vi "RangeCases.vi"() -> ()   [LabVIEW 2019]
panel:
  in  "Numeric 2":u8
  in  "Numeric":u8
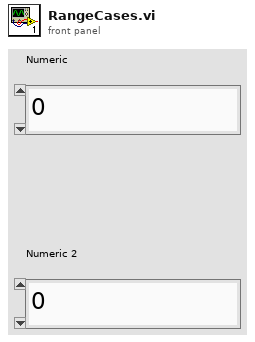
[diagram p1: front panel]
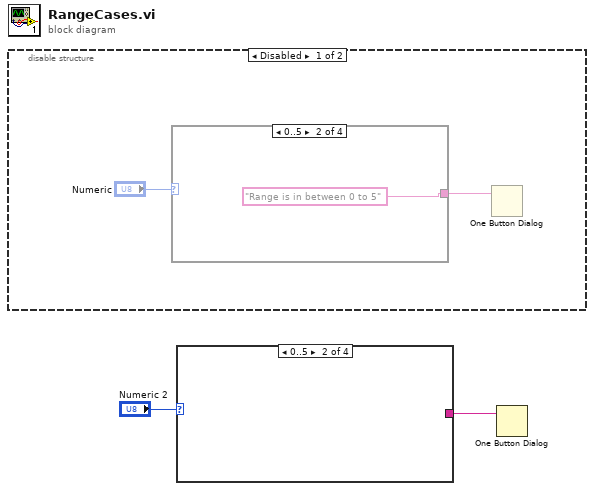
[diagram p0: block diagram]
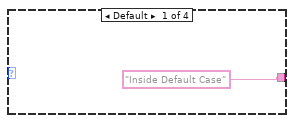
[diagram p2: hidden frame]
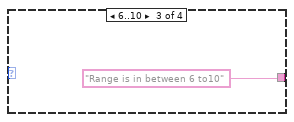
[diagram p3: hidden frame]
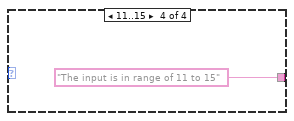
[diagram p4: hidden frame]
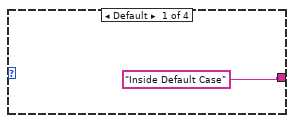
[diagram p6: hidden frame]
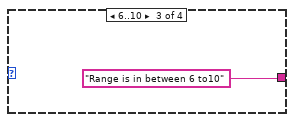
[diagram p7: hidden frame]
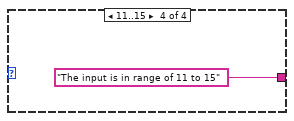
[diagram p8: hidden frame]
diagram:
  n1 = disable-structure shown="Disabled" {
    frame Disabled {
      n2 = case shown="0..5" "Numeric" {
        tunnel: ["Inside Default Case" ("message") "Range is in between 0 to 5" ("message") "Range is in between 6 to10" ("message") "The input is in range of 11 to 15" ("message")] -> w3
        frame Default {
        }
        frame 0..5 {
        }
        frame 6..10 {
        }
        frame 11..15 {
        }
      }
      n3 = One Button Dialog(message=w3) -> ()  [unwired: 1 in, 1 out]
    }
    frame Enabled {
    }
  }
  n4 = case shown="0..5" "Numeric 2" {
    tunnel: ["Inside Default Case" ("message") _ "Range is in between 6 to10" ("message") "The input is in range of 11 to 15" ("message")] -> w2
    frame Default {
    }
    frame 0..5 {
    }
    frame 6..10 {
    }
    frame 11..15 {
    }
  }
  n5 = One Button Dialog(message=w2) -> ()  [unwired: 1 in, 1 out]
